vi "DIP Switch - Read-SubVI.vi"(8 "error in (no error)":errorcluster, 11 "AI Ref In":T1) -> (0 "error out":errorcluster, 3 "DIP State":T10)   [LabVIEW 2021]
uses:
  Main - States_SubVI.ctl
  <vilib>/myRIO/Instrument Drivers/Onboard IO/AI/typedefs/AI Reference.ctl
  <vilib>/myRIO/Common/Instrument Driver Framework/Utilities/typedefs/myRIO Generic Hardware Reference.ctl
  <vilib>/myRIO/Common/Instrument Driver Framework/Utilities/typedefs/Hardware Version Enum.ctl
  <vilib>/myRIO/Common/Instrument Driver Framework/Utilities/typedefs/myRIO v1.0 Reference.ctl
  <vilib>/myRIO/Common/Instrument Driver Framework/Utilities/typedefs/Generic FPGA Reference.ctl
  <vilib>/myRIO/Common/Instrument Driver Framework/myRIO v1.0/AI/typedefs/AI Channels List.ctl
  <vilib>/myRIO/Common/Instrument Driver Framework/myRIO v1.0/AI/typedefs/AI Channels Enum.ctl
  <vilib>/myRIO/Common/Instrument Driver Framework/Utilities/typedefs/Analog Scaling Constants List.ctl
  <vilib>/myRIO/Common/Instrument Driver Framework/Utilities/typedefs/Analog Scaling Constants.ctl
  <vilib>/Utility/error.llb/Error Cluster From Error Code.vi
  <vilib>/myRIO/Common/Instrument Driver Framework/myRIO v1.0/AI/vis/myRIO v1.0 Read AI.vi
  <vilib>/myRIO/Instrument Drivers/Onboard IO/AI/AI.lvlib
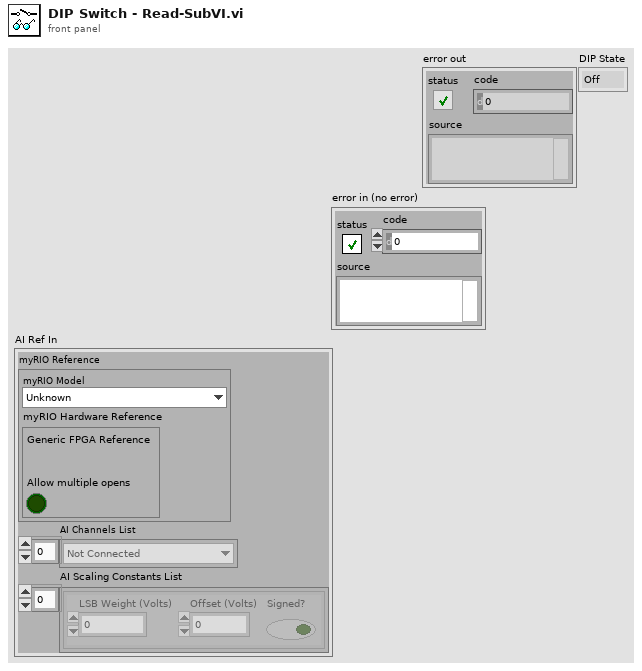
[diagram p1: front panel]
types:
  T1 = typedef "AI.lvlib/AI Reference.ctl" = cluster{"myRIO Reference":T2, "AI Channels List":T6, "AI Scaling Constants List":T8}
  T2 = typedef "myRIO Generic Hardware Reference.ctl" = cluster{"myRIO Model":T3, "myRIO Hardware Reference":T4}
  T3 = typedef "Hardware Version Enum.ctl" = enum16{"Unknown", "myRIO-1900", "myRIO-1950", "roboRIO", "NI ELVIS RIO CM", "ELVIS III"}
  T4 = typedef "myRIO v1.0 Reference.ctl" = cluster{"Generic FPGA Reference":T5, "Allow multiple opens":bool}
  T5 = typedef "Generic FPGA Reference.ctl" = refnum<k20>
  T6 = typedef "AI Channels List.ctl" = T7[]
  T7 = typedef "AI Channels Enum.ctl" = enum16{"Not Connected", "AudioIn/Left", "AudioIn/Right", "C/AI0", "C/AI1", "A/AI0", "A/AI1", "A/AI2", "A/AI3", "A/AI4", "A/AI5", "A/AI6", "A/AI7", "B/AI0", "B/AI1", "B/AI2", "B/AI3", "B/AI4", "B/AI5", "B/AI6", "B/AI7", "AI/AI0", "AI/AI1", "AI/AI2", "AI/AI3", "A/AI0 (DIFF)", "A/AI1 (DIFF)", "A/AI2 (DIFF)", "A/AI3 (DIFF)", "B/AI0 (DIFF)", "B/AI1 (DIFF)", "B/AI2 (DIFF)", "B/AI3 (DIFF)"}
  T8 = typedef "Analog Scaling Constants List.ctl" = T9[]
  T9 = typedef "Analog Scaling Constants.ctl" = cluster{"LSB Weight (Volts)":dbl, "Offset (Volts)":dbl, "Signed?":bool}
  T10 = typedef "Main - States_SubVI.ctl" = enum16{"Off", "Record", "Upload", "Shutdown", "Error"}
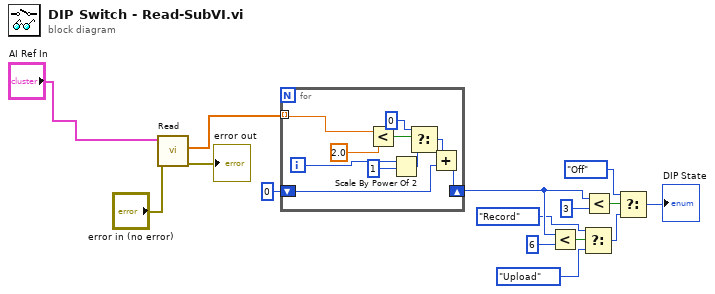
[diagram p0: block diagram]
diagram:
  n1 = call <vilib>:"Read.vi"("error in (no error)"="error in (no error)", "AI Ref In"="AI Ref In") -> ("error out"=→"error out":errorcluster, "Values"=w14:dbl[])  [unwired: 7 in, 1 out]
  n2 = for {
    tunnel: w14 -> [w16] mode=indexing
    shift-right: [w17] -> w5
    shift-left: 0 ("f") -> [w18]
    i -> [w21]
    n3 = Less?(x=w16, y=2.0) -> (x < y?=w25:bool)
    n4 = Scale By Power Of 2(n=w21, x=1) -> (x*2^n=w20:i32)
    n5 = Select(t=0 ("f"), s=w25, f=w20) -> (s? t:f=w19:i32)
    n6 = Add(x=w19, y=w18) -> (x+y=w17:i32)
  }
  n7 = Less?(x=w5, y=6) -> (x < y?=w6:bool)
  n8 = Select(t=Main_-_States_SubVI."Record" ("Enum"), s=w6, f=Main_-_States_SubVI."Upload" ("Enum")) -> (s? t:f=w8:T10)
  n9 = Less?(x=w5, y=3) -> (x < y?=w11:bool)
  n10 = Select(t=Main_-_States_SubVI."Off" ("Enum"), s=w11, f=w8) -> (s? t:f=→"DIP State":T10)
